vi "BooleanDataType.vi"() -> ()   [LabVIEW 2019]
panel:
  out "IndBool":bool
  in  "flag":bool
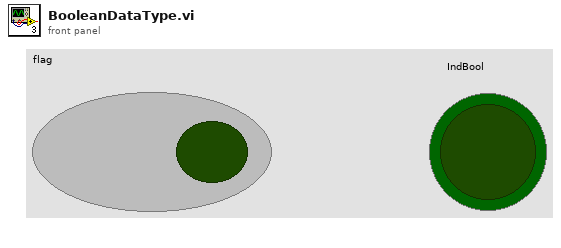
[diagram p1: front panel]
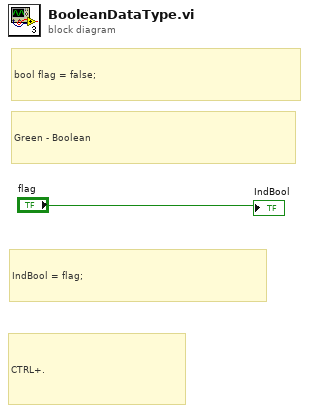
[diagram p0: block diagram]
diagram:
  # "CTRL+."
  # "IndBool = flag;"
  # "Green - Boolean"
  # "bool flag = false;"
  "IndBool" <- "flag"
